vi "Create_K7DRAMFIFO.vi"(8 "Requested # of Elements":u32, 10 "DRAM Bank Ref 2":refnum<k21>, 11 "DRAM Bank Ref 1":refnum<k21>) -> (3 "DRAM FIFO Ref Out":refnum<class "K7 DRAM FIFO.lvclass">)   [LabVIEW 2014, in "K7 DRAM FIFO.lvclass"]
doc: "Creates a reference to a DRAM FIFO on the block diagram.\n\n<B>Inputs</B>\n<B>Memory Refnum</B> specifies the memory item that the FIFO will stream data through. See detailed help for more information.\n<B>Requested # of Elements</B> is the number of requested elements in the memory item used by the FIFO. This will define how deep the FIFO is.\n\n<B>Outputs</B>\n<B>DRAM FIFO Ref Out</B> is the reference to the DRAM FIFO\n\n<B>Detailed Help</B>\nThe Memory Refnum must point to memory item that uses a data type that is a custom control defined by the control located at <LabVIEW>\\instr.lib\\_niInstr\\Memory\\v1\\FPGA\\Memory\\Public\\U512.ctl. \n\nThe Memory Refnum must point to memory item that is implemented using DRAM. \n\nIf the DRAM FIFO is executed in simulation mode, the Memory Refnum must point to a memory item that allocates 1MB of memory or less. Simulating more than 1MB of DRAM memory may result in an error. \n\nThe Requested # of Elements should be equal to the number shown in the properties page of the memory item. When naming the memory item, consider appending the number of elements requested by the memory item to the name of the memory item to avoid using the wrong number."
uses:
  K7 DRAM FIFO.lvclass
  K7 DRAM FIFO.lvclass/K7 DRAM FIFO.ctl
  <instrlib>/_niInstr/Memory/v1/FPGA/DRAM/Private/Create U128x2.vi
  <vilib>/rvi/DataTransferAndStorage/Container/Common/niFpgaContainerGetUniqueNameForEmu.vi
  <vilib>/rvi/DataTransferAndStorage/Container/Common/niFpgaContainerSetEmuInfo.vi
  <vilib>/rvi/eio/common/nirviEmuReportErrorAndStop.vi
  <vilib>/rvi/LocalResourceManager/LocalResourceManager.xnode
  <instrlib>/_niInstr/Memory/v1/FPGA/DRAM/niInstr Memory DRAM v1 FPGA.lvclass
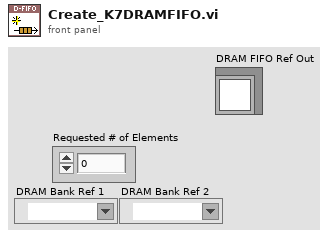
[diagram p1: front panel]
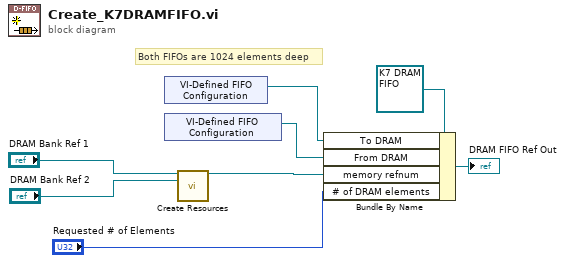
[diagram p0: block diagram]
diagram:
  # "Both FIFOs are 1024 elements deep"
  n1 = xnode "VI-Defined FIFO Configuration"() -> ("FIFO Out"=w4:refnum<k21>)
  n2 = xnode "VI-Defined FIFO Configuration"() -> ("FIFO Out"=w5:refnum<k21>)
  n3 = call-poly <instrlib>:"Create Resources.vi"("memory 1"="DRAM Bank Ref 1", "memory 2"="DRAM Bank Ref 2") -> ("memory out"=w6:refnum<class "niInstr Memory DRAMx2 v1 FPGA.lvclass">)  [unwired: 13 in]
  n4 = Bundle By Name(cluster=refnum<class "K7 DRAM FIFO.lvclass"> refnum ("K7 DRAM FIFO.lvclass 2"), "To DRAM"=w4, "From DRAM"=w5, "memory refnum"=w6, "# of DRAM elements"="Requested # of Elements") -> (→"DRAM FIFO Ref Out":refnum<class "K7 DRAM FIFO.lvclass">)
